vi "Get UI Details.vi"(8 "error in (no error)":errorcluster) -> (0 "error out":errorcluster, 2 "UI Details":T1[](array[typedef]))   [LabVIEW 2020, in "MeasurementLink Measurement Template.lvlib"]
uses:
  MeasurementLink Measurement Template.lvlib
  MeasurementLink Measurement Server/Helpers/TypeDefs/UI Information.ctl
  Measurement UI.vi
  MeasurementLink Measurement Server/MeasurementLink Measurement Server.lvlib
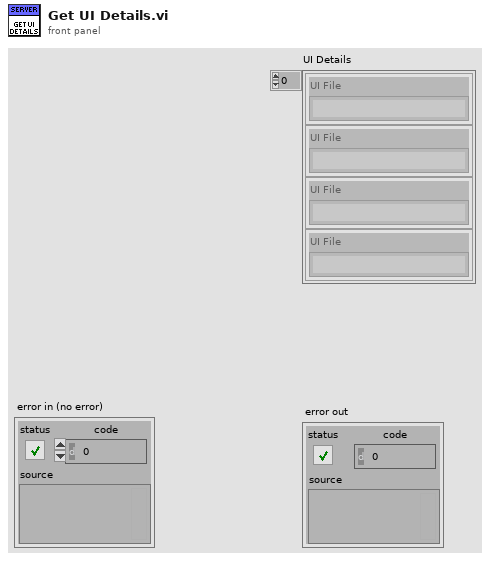
[diagram p1: front panel]
types:
  T1 = typedef "MeasurementLink Measurement Server.lvlib/UI Information.ctl" = cluster{"UI File":string}
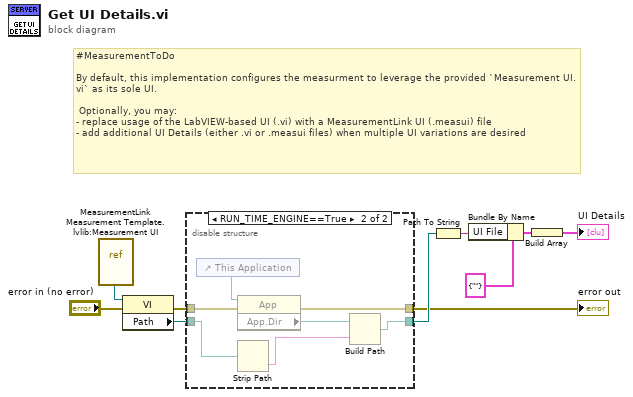
[diagram p0: block diagram]
diagram:
  # "#MeasurementToDo\n\nBy default, this implementation configures the measurment to leverage the provided `Measurement UI.vi` as its sole UI.\n\n Optionally, you may:\n- replace usage of the LabVIEW-based UI (.vi) with a MeasurementLink UI (.measui) file\n- add additional UI Details (either .vi or .measui files) when multiple UI variations are desired"
  n1 = vi-ref "MeasurementLink Measurement Template.lvlib:Measurement UI.vi"() -> (w4:refnum<vi>)
  n2 = property class="VI"(reference=w4, error in="error in (no error)") -> (error out=w2:errorcluster, "Path"=w1:path)  [unwired: 1 out]
  n3 = disable-structure shown="RUN_TIME_ENGINE==True" {
    disable-tunnel: [w11 w13] -> w6
    disable-tunnel: w2 -> [w12 w18]
    disable-tunnel: [w12 w17] -> w5
    disable-tunnel: w1 -> [w11 w15]
    frame condition #0 (active) {
    }
    frame condition #1 {
      n4 = control-ref of="This Application"() -> (w19:refnum<vi>)
      n5 = property class="App"(reference=w19, error in=w18) -> (error out=w17:errorcluster, "App.Dir"=w16:path)  [unwired: 1 out]
      n6 = Strip Path(path=w15) -> (name=w14:string)  [unwired: 1 out]
      n7 = Build Path(base path=w16, name or relative path=w14) -> (appended path=w13:path)
    }
  }
  "error out" <- w5
  n8 = Path To String(path=w6) -> (string=w7:string)
  n9 = Bundle By Name(cluster=T1 {"UI File"=""} ("UI Information"), "UI File"=w7) -> (w9:T1)
  n10 = Build Array(w9) -> (→"UI Details":T1[])
